vi "SubVI_ParseCommand_Auto.vi"(11 "String":string="foward,90") -> (3 "array":string[](array[string]))   [LabVIEW 2017]
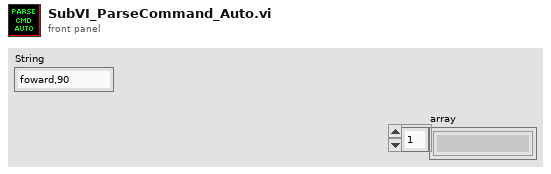
[diagram p1: front panel]
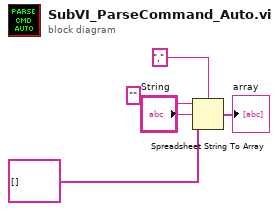
[diagram p0: block diagram]
diagram:
  n1 = Spreadsheet String To Array(delimiter (Tab)=",", format string="", spreadsheet string="String", array type (2D Dbl)=string[] [] ("String Array")) -> (array=→"array":string[])
